vi "sbrio_sys.vi"() -> ()   [LabVIEW 2014]
uses:
  <vilib>/FPGAPlugInAG/sbRIO-9636/niLvFpga_Open_sbRIO-9636.vi
  <vilib>/rvi/interface/common/dynamic/niFpgaDynamicAddResources.vi
  <vilib>/Utility/error.llb/Error Cluster From Error Code.vi
  <vilib>/rvi/errors/niLvFpgaAdjustHostInterfaceError.vi
  <vilib>/rvi/interface/nirviOpenFPGA/nirviOpenFPGA.xnode
  FPGA Bitfiles/proj_FPGATarget_fpga_6iQAp21sY34.lvbitx
  fpga.vi
  <vilib>/rvi/interface/nirviReadWriteControl/nirviReadWriteControl.xnode
  NiFpgaLv.dll
  <vilib>/rvi/interface/Simulation/niFpgaSimulationCallBeginRW.vi
panel:
  out "Waveform Chart":dbl(graph)
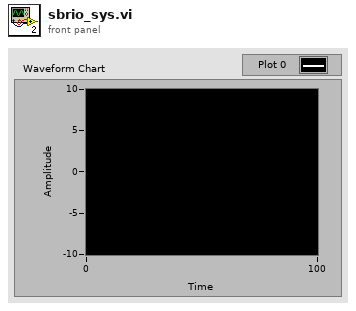
[diagram p1: front panel]
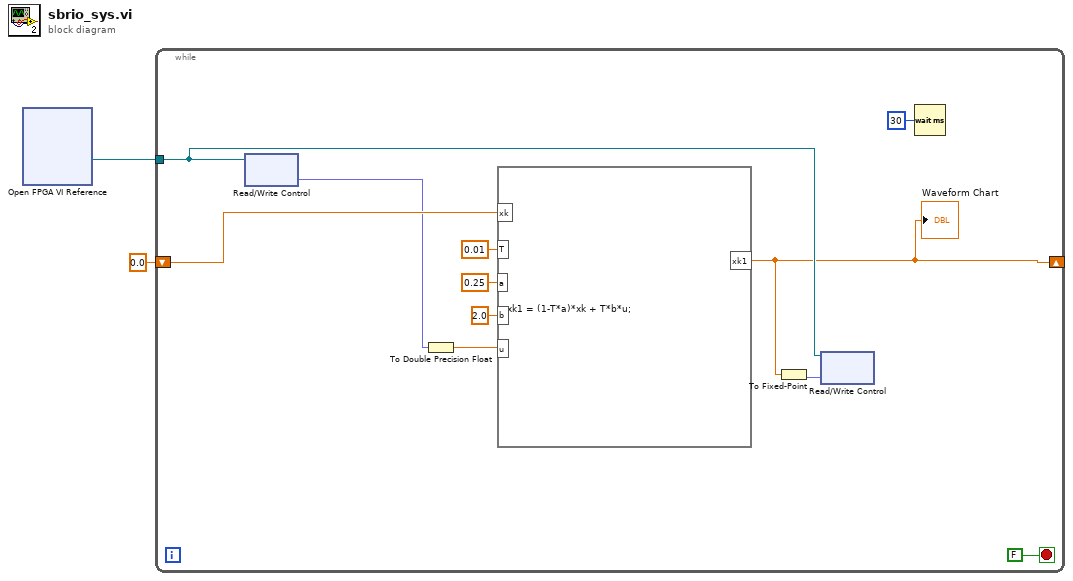
[diagram p0: block diagram]
diagram:
  n1 = xnode "Open FPGA VI Reference"() -> ("FPGA VI Reference Out"=w1:refnum<k20>)  [unwired: 2 in, 1 out]
  n2 = while {
    shift-right: [w4] -> _
    shift-left: 0.0 ("xk1") -> [w13]
    tunnel: w1 -> [w5]
    stop <- FALSE stop-if-true
    n3 = xnode "Read/Write Control"("FPGA VI Reference In"=w5) -> ("AI0"=w7:fxp<+/-,24,5>)  [unwired: 1 in, 2 out]
    n4 = To Double Precision Float(number=w7) -> (double precision float=w8:dbl)
    n5 = formula code="xk1 = (1-T*a)*xk + T*b*u;"("xk"=w13, "T"=0.01 ("input variable"), "a"=0.25 ("input variable"), "b"=2.0 ("input variable"), "u"=w8) -> ("xk1"=w4:dbl)
    "Waveform Chart" <- w4
    n6 = To Fixed-Point(number=w4) -> (fixed-point=w6:fxp<+/-,32,16>)  [unwired: 1 in]
    n7 = xnode "Read/Write Control"("FPGA VI Reference In"=w5, "AO0"=w6) -> ()  [unwired: 1 in, 2 out]
    n8 = Wait (ms)(milliseconds to wait=u32 30) -> ()  [unwired: 1 out]
  }
